vi "GUIAS POTÊNCIA VS VELOCIDADE.vi"() -> ()   [LabVIEW 2014]
uses:
  <vilib>/Platform/TimedLoop/XDataNode/timing_clust.ctl
  <vilib>/Platform/TimedLoop/XDataNode/nitl_modes.ctl
  <vilib>/Platform/TimedLoop/XDataNode/wakeup.ctl
  <vilib>/Instr/_visa.llb/VISA Configure Serial Port (Instr).vi
  <vilib>/Platform/TimedLoop/XDataNode/XDataNode.xnode
  <userlib>/Newport ESP301/Newport ESP301.lvlib
  <vilib>/Platform/TimedLoop/XDataNode/XDNodeRunTimeDep.lvlib
panel:
  in  "Refresh Button":bool
  out "XY Graph":cluster{dbl[], dbl[]}(graph)={[0.0, 0.0, 0.0, 0.0, 0.0, 0.0, 0.0, 0.0, 0.0, 0.0, 0.0, 0.0, 0.0, 0.0, 0.0, 0.0, 0.0, 0.0, 0.0, 0.0, 0.0, 0.0, 0.0, 0.0, 0.0, 0.0, 0.0, 0.0, 0.0, 0.0, 0.0, 0.0, 0.0, 0.0, 0.0, 0.0, 0.0, 0.0, 0.0, 0.0, 0.0, 0.0, 0.0, 0.0, 0.0, 0.0, 0.0, 0.0, 0.0, 0.0, 0.0, 0.0, 0.0, 0.0, 0.0, 0.0, 0.0, 0.0, 0.0, 0.0, 0.0, 0.0, 0.0, 0.0, 0.0, 0.0, 0.0, 0.0, 0.0, 0.0, 0.0, 0.0, 0.0, 0.0, 0.0, 0.0], [4600.0, 4600.0, 4600.0, 4600.0, 4600.0, 4600.0, 4600.0, 4600.0, 4600.0, 4600.0, 4600.0, 4600.0, 4600.0, 4600.0, 4600.0, 4600.0, 4600.0, 4600.0, 4600.0, 4600.0, 4600.0, 4600.0, 4600.0, 4600.0, 4600.0, 4600.0, 4600.0, 4690.0, 4802.5, 4800.5, 4799.5, 4799.5, 4799.5, 4800.0, 4800.0, 4800.0, 4800.0, 4800.0, 4800.0, 4800.0, 4800.0, 4800.0, 4800.0, 4800.0, 4995.5, 5001.5, 5000.5, 5000.0, 5000.0, 4999.5, 4999.5, 5000.0, 5000.0, 5000.0, 5000.0, 5000.0, 5000.0, 5000.0, 5000.0, 5000.0, 5000.0, 5000.0, 5000.0, 5000.0, 5000.0, 5000.0, 5000.0, 5000.0, 5000.0, 5000.0, 5000.0, 5000.0, 5000.0, 5000.0, 5000.0, 5000.0]}
  out "Y (um)":dbl format="%.1f"
  out "X (mm)":dbl format="%.2g"
  out "PROGRESSÃO":i32
  in  "DistGrupos":bool
  in  "dGroup":dbl=200.0
  in  "dGuia":dbl=100.0 format="%#_6f"
  in  "Iniciar":bool
  in  "Stop Button":bool
  in  "L":dbl=3.0 format="%.1f"
  in  "VELOCIDADES":dbl[](array[numeric])=[1.0, 5.0, 10.0, 20.0]
  in  "N_veloc":dbl=4.0
  # "Número de velocidades\npor potência"
  # "TAMANHO DA AMOSTRA (mm)"
  # "DISTÂNCIA ENTRE GUIAS (um)"
  # "DISTÂNCIA ENTRE GRUPOS (um)"
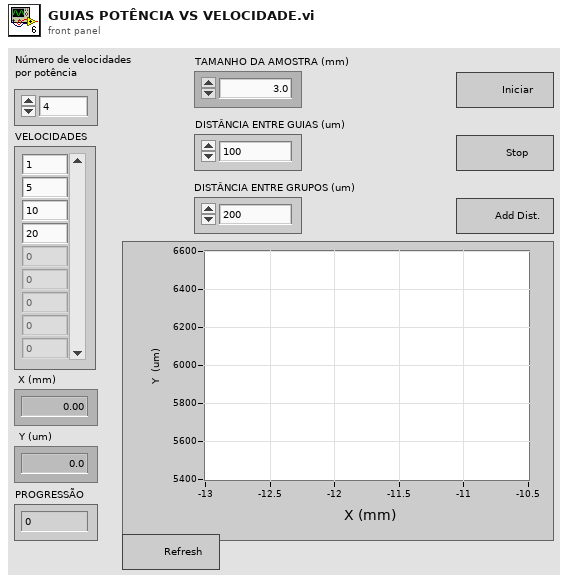
[diagram p1: front panel]
types:
  T1 = typedef "XDNodeRunTimeDep.lvlib/timing_clust.ctl" = cluster{"Expected End [f-1]":u64, "Actual End [f-1]":u64, "Finished Late? [f-1]":bool, "Expected End [i-1]":u64, "Actual End [i-1]":u64, "Finished Late? [i-1]":bool, "Expected Start [i]":u64, "Actual Start [i]":u64, "Expected Start [f]":u64, "Actual Start [f]":u64, "Source Name":string, "Structure Name":string, "Period":i64, "Deadline":i64, "Offset":i64, "Start":i64, "Priority":i32, "Timeout":i32, "Mode":T2, "Wakeup Reason":T3, "Error":errorcluster, "Source Type":string, "Secondary Source Type":string, "Global End Time":u64, "Global Start Time":u64, "Frame Duration":u64, "Iteration Duration":u64, "Assigned CPU":i32, "I/O Scan Engine Mode":u32}
  T2 = typedef "XDNodeRunTimeDep.lvlib/nitl_modes.ctl" = enum32{"No Change", "Process missed periods, maintain original phase", "Discard missed periods, maintain original phase", "Process missed periods, ignore original phase", "Discard missed periods, ignore original phase"}
  T3 = typedef "XDNodeRunTimeDep.lvlib/wakeup.ctl" = enum32{"Normal", "Aborted", "Asynchronous wakeup", "Timing source error", "Timed loop error", "Timeout"}
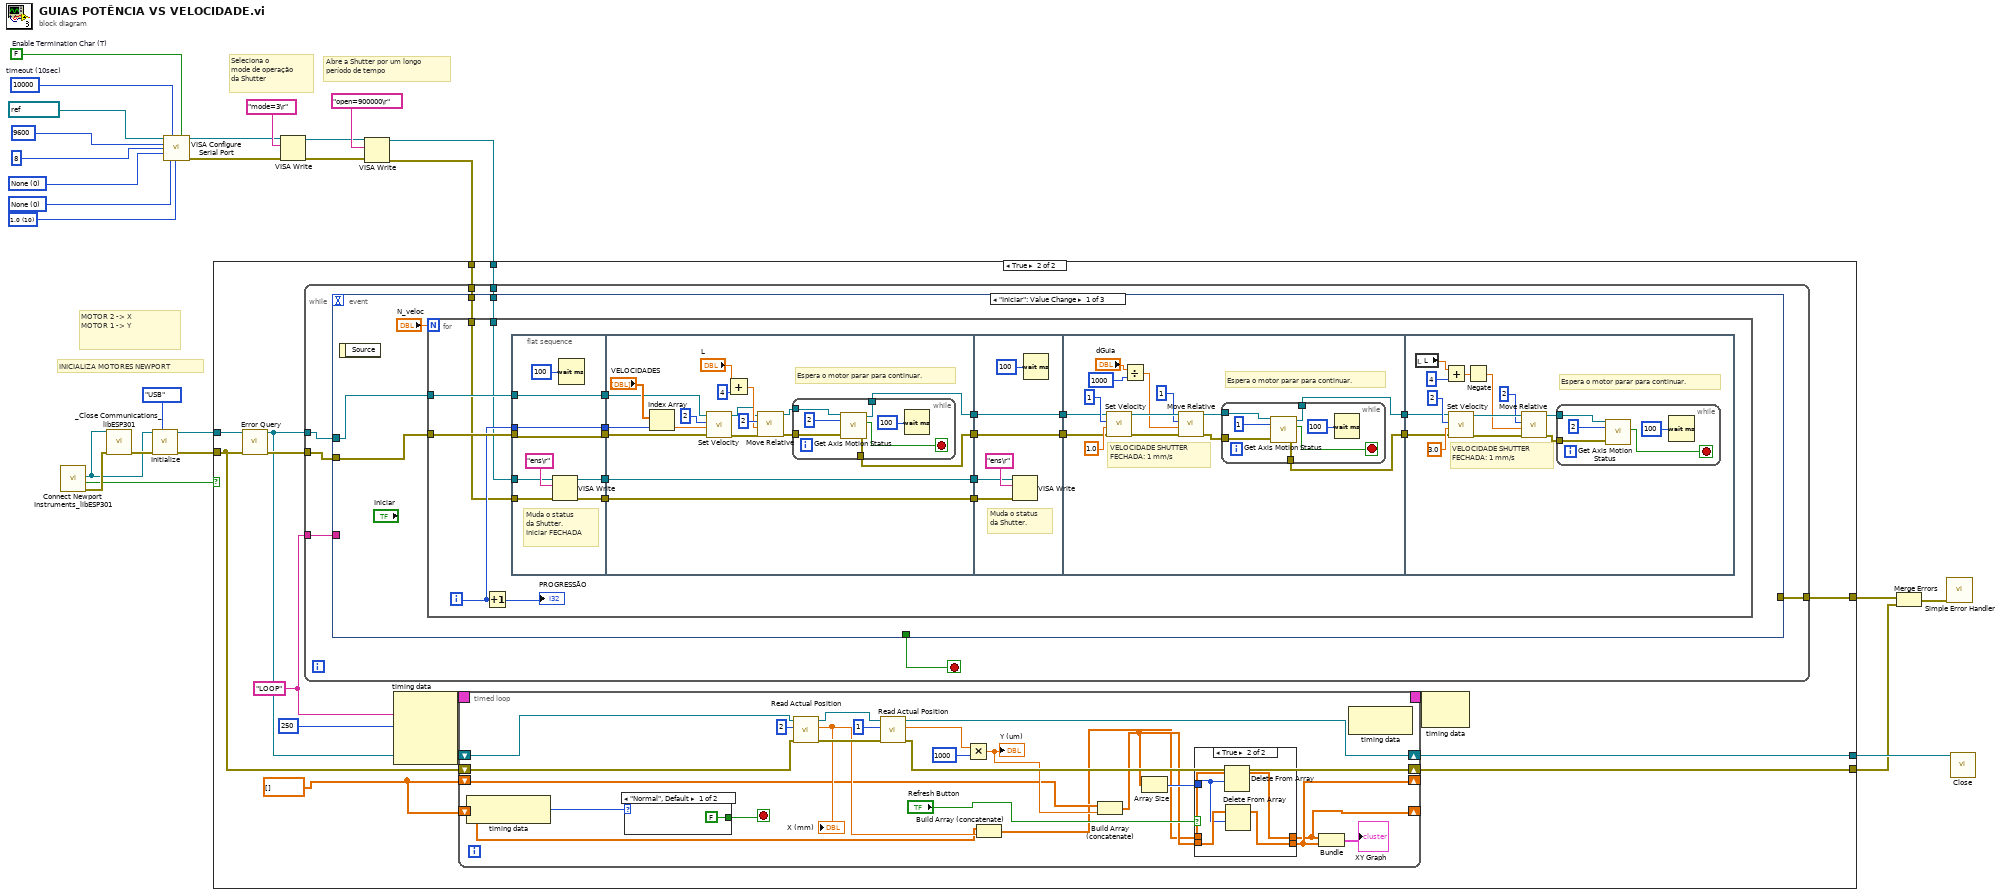
[diagram p0: block diagram]
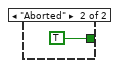
[diagram p4: hidden frame]
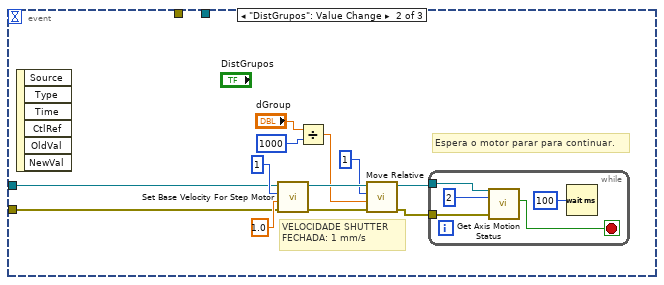
[diagram p5: hidden frame]
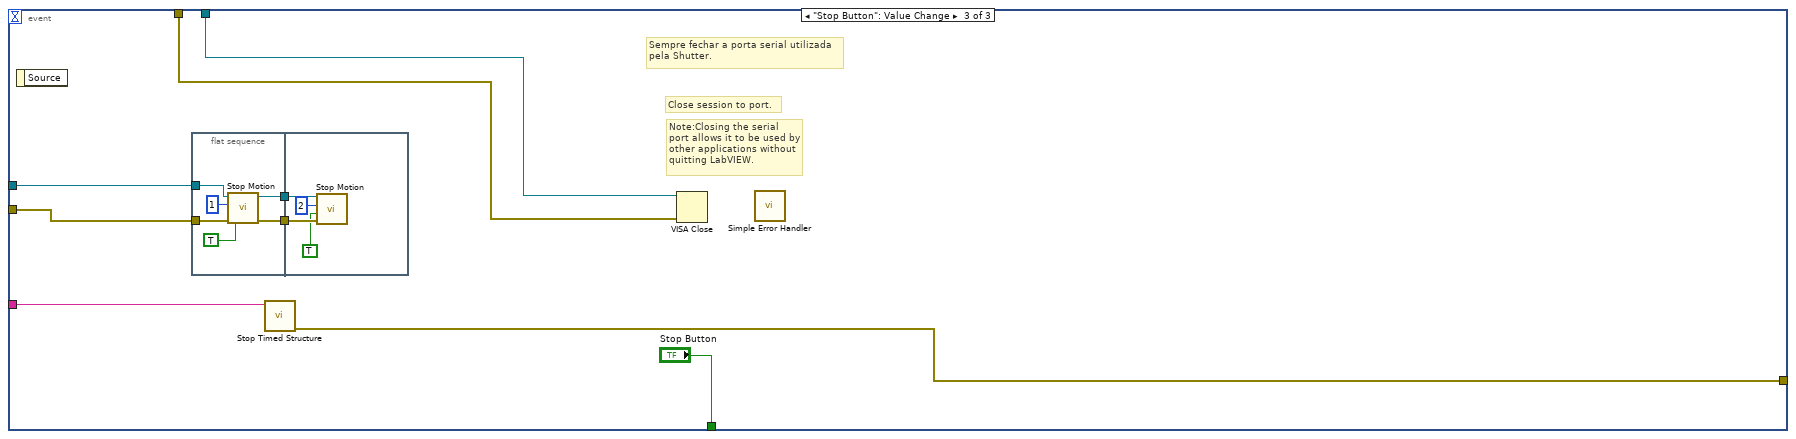
[diagram p6: hidden frame]
diagram:
  w15 = u16 0 items=["None", "Odd", "Even", "Mark", "Space"] ("parity")
  w18 = u16 10 items=["1.0"=10, "1.5"=15, "2.0"=20] ("stop bits")
  w19 = u16 0 items=["None"=0, "XON/XOFF"=1, "RTS/CTS"=2, "DTR/DSR"=4] ("flow control")
  w17 = FALSE  # Enable Termination Char (T)
  w16 = u32 10000  # timeout (10sec)
  # "MOTOR 2 -> X\nMOTOR 1 -> Y"
  # "Abre a Shutter por um longo\nperíodo de tempo"
  # "Seleciona o \nmode de operação\nda Shutter"
  # "INICIALIZA MOTORES NEWPORT"
  n1 = call <userlib>:"Connect Newport Instruments_libESP301.vi"() -> ("error (duplicate)"=w25:errorcluster, "Connected"=w23:bool, "VISA resource name (duplicate)"=w24:refnum<visa-resource-name>)  [unwired: 7 in, 2 out]
  n2 = call <userlib>:"_Close Communications_libESP301.vi"("Instrument Channel"=w24, "error in (no error)"=w25) -> ("error out"=w27:errorcluster)  [unwired: 13 in]
  n3 = call <userlib>:"Initialize.vi"("VISA resource name"=w24, "error in (no error)"=w27, "Serial Link (RS232)"=enum16{"RS232", "USB"}."USB") -> ("VISA resource name out"=w21:refnum<visa-resource-name>, "error out"=w22:errorcluster)  [unwired: 6 in]
  n4 = call-poly "VISA Configure Serial Port"("VISA resource name"=refnum<visa-resource-name> "COM6", "timeout (10sec)"=w16, "Enable Termination\nChar (T)"=w17, "baud rate (9600)"=u32 9600 ("baud rate"), "data bits (8)"=u16 8 ("data bits"), "parity (0:none)"=w15, "stop bits (10: 1 bit)"=w18, "flow control (0:none)"=w19) -> ("VISA resource name out"=w11:refnum<visa-resource-name>, "error out"=w10:errorcluster)  [unwired: 6 in]
  n5 = VISA Write(VISA resource name=w11, write buffer="mode=3\r", error in (no error)=w10) -> (VISA resource name out=w8:refnum<visa-resource-name>, error out=w7:errorcluster)  [unwired: 1 out]
  n6 = VISA Write(VISA resource name=w8, write buffer="open=900000\r", error in (no error)=w7) -> (VISA resource name out=w2:refnum<visa-resource-name>, error out=w1:errorcluster)  [unwired: 1 out]
  n7 = case shown="True" w23 {
    tunnel: w22 -> [w28 w39]
    tunnel: w21 -> [w29 w43]
    tunnel: [w29 w36] -> w6
    tunnel: [w28 w35] -> w4
    tunnel: [_ w33] -> w5
    tunnel: w2 -> [_ w32]
    tunnel: w1 -> [_ w31]
    frame False {
    }
    frame True {
      w30 = dbl[] []
      w34 = "LOOP" ("Structure Name")
      n8 = call <userlib>:"Error Query.vi"("error in (no error)"=w39, "VISA resource name"=w43) -> ("error out"=w42:errorcluster, "VISA resource name out"=w38:refnum<visa-resource-name>)  [unwired: 2 in, 2 out]
      n9 = while {
        tunnel: w38 -> [w90]
        tunnel: w42 -> [w89]
        tunnel: w34 -> [w87]
        tunnel: [w86] -> w33
        tunnel: w32 -> [w85]
        tunnel: w31 -> [w84]
        stop <- w88 stop-if-true
        n10 = event shown="[0] \"Iniciar\": Value Change" {
          selector: _ -> [_ _ _]
          dyn-events: _ -> [_ _ _]
          timeout: _ -> [_ _ _]
          tunnel: w90 -> [w93 w198 w217]
          tunnel: w89 -> [w94 w197 w216]
          tunnel: [_ _ "Stop Button"] -> w88
          tunnel: w87 -> [_ _ w214]
          tunnel: [_ _ w213] -> w86
          tunnel: w85 -> [w92 _ w212]
          tunnel: w84 -> [w91 _ w211]
          event "Iniciar": Value Change {
            n11 = event-data() -> ()  [unwired: 1 in, 1 out]
            n12 = for {
              N: "N_veloc" -> [_]
              tunnel: w94 -> [w114]
              tunnel: w93 -> [w113]
              tunnel: w92 -> [w98]
              tunnel: w91 -> [w97]
              i -> [w106]
              n13 = Increment(x=w106) -> (x+1=→"PROGRESSÃO":i32)
              n14 = flat-sequence {
                tunnel: w113 -> [w121]
                tunnel: w114 -> [w122]
                tunnel: w106 -> [w123]
                tunnel: [w123] -> w112
                tunnel: [w122] -> w111
                tunnel: [w121] -> w110
                tunnel: [w118] -> w109
                tunnel: [w117] -> w108
                tunnel: w98 -> [w116]
                tunnel: w97 -> [w115]
                tunnel: w112 -> [w141]
                tunnel: w111 -> [w129]
                tunnel: w110 -> [w128]
                tunnel: [w133] -> w104
                tunnel: w109 -> [w133]
                tunnel: w108 -> [w132]
                tunnel: [w132] -> w103
                tunnel: [w125] -> w101
                tunnel: [w124] -> w99
                tunnel: w104 -> [w152]
                tunnel: w103 -> [w151]
                tunnel: [w150] -> w102
                tunnel: w101 -> [w150]
                tunnel: [w149] -> w100
                tunnel: w99 -> [w149]
                tunnel: [w156] -> w107
                tunnel: w102 -> [w160]
                tunnel: w100 -> [w159]
                tunnel: [w155] -> w96
                tunnel: w107 -> [w179]
                tunnel: w96 -> [w178]
                frame #0 {
                  # "Muda o status\nda Shutter.\nIniciar FECHADA"
                  n15 = VISA Write(VISA resource name=w116, write buffer="ens\r", error in (no error)=w115) -> (VISA resource name out=w118:refnum<visa-resource-name>, error out=w117:errorcluster)  [unwired: 1 out]
                  n16 = Wait (ms)(milliseconds to wait=u32 100) -> ()  [unwired: 1 out]
                }
                frame #1 {
                  # "Espera o motor parar para continuar."
                  n17 = Index Array(array="VELOCIDADES", index=w141) -> (element=w134:dbl)
                  n18 = call <userlib>:"Set Velocity.vi"("error in (no error)"=w129, "Velocity (units/s)"=w134, "Axis (1)"=2, "VISA resource name"=w128) -> ("error out"=w130:errorcluster, "VISA resource name out"=w131:refnum<visa-resource-name>)  [unwired: 2 in]
                  n19 = Add(x="L", y=4) -> (x+y=w137:dbl)
                  n20 = call <userlib>:"Move Relative.vi"("error in (no error)"=w130, "Position (0 units)"=w137, "Axis (1)"=2, "VISA resource name"=w131) -> ("error out"=w127:errorcluster, "VISA resource name out"=w126:refnum<visa-resource-name>)  [unwired: 2 in]
                  n21 = while {
                    tunnel: [w145] -> w124
                    tunnel: [w144] -> w125
                    tunnel: w127 -> [w143]
                    tunnel: w126 -> [w142]
                    stop <- w147 stop-if-true
                    n22 = call <userlib>:"Get Axis Motion Status.vi"("error in (no error)"=w143, "Axis (1)"=2, "VISA resource name"=w142) -> ("error out"=w144:errorcluster, "Motion Done"=w147:bool, "VISA resource name out"=w145:refnum<visa-resource-name>)  [unwired: 2 in]
                    n23 = Wait (ms)(milliseconds to wait=u32 100) -> ()  [unwired: 1 out]
                  }
                }
                frame #2 {
                  # "Muda o status\nda Shutter."
                  n24 = VISA Write(VISA resource name=w152, write buffer="ens\r", error in (no error)=w151) -> ()  [unwired: 3 out]
                  n25 = Wait (ms)(milliseconds to wait=u32 100) -> ()  [unwired: 1 out]
                }
                frame #3 {
                  # "Espera o motor parar para continuar."
                  # "VELOCIDADE SHUTTER\nFECHADA: 1 mm/s"
                  n26 = call <userlib>:"Set Velocity.vi"("error in (no error)"=w160, "Velocity (units/s)"=1.0 ("Base Velocity (0 units/s)"), "Axis (1)"=1, "VISA resource name"=w159) -> ("error out"=w167:errorcluster, "VISA resource name out"=w166:refnum<visa-resource-name>)  [unwired: 2 in]
                  n27 = Divide(x="dGuia", y=1000) -> (x/y=w161:dbl)
                  n28 = call <userlib>:"Move Relative.vi"("error in (no error)"=w167, "Position (0 units)"=w161, "Axis (1)"=1, "VISA resource name"=w166) -> ("error out"=w157:errorcluster, "VISA resource name out"=w158:refnum<visa-resource-name>)  [unwired: 2 in]
                  n29 = while {
                    tunnel: [w172] -> w156
                    tunnel: [w171] -> w155
                    tunnel: w157 -> [w170]
                    tunnel: w158 -> [w169]
                    stop <- w174 stop-if-true
                    n30 = call <userlib>:"Get Axis Motion Status.vi"("error in (no error)"=w170, "Axis (1)"=1, "VISA resource name"=w169) -> ("error out"=w171:errorcluster, "Motion Done"=w174:bool, "VISA resource name out"=w172:refnum<visa-resource-name>)  [unwired: 2 in]
                    n31 = Wait (ms)(milliseconds to wait=u32 100) -> ()  [unwired: 1 out]
                  }
                }
                frame #4 {
                  # "Espera o motor parar para continuar."
                  # "VELOCIDADE SHUTTER\nFECHADA: 1 mm/s"
                  n32 = local read "L"() -> (w182:dbl)
                  n33 = Add(x=w182, y=4) -> (x+y=w181:dbl)
                  n34 = call <userlib>:"Set Velocity.vi"("error in (no error)"=w178, "Velocity (units/s)"=3.0 ("Base Velocity (0 units/s)"), "Axis (1)"=2, "VISA resource name"=w179) -> ("error out"=w187:errorcluster, "VISA resource name out"=w186:refnum<visa-resource-name>)  [unwired: 2 in]
                  n35 = Negate(x=w181) -> (-x=w180:dbl)
                  n36 = call <userlib>:"Move Relative.vi"("error in (no error)"=w187, "Position (0 units)"=w180, "Axis (1)"=2, "VISA resource name"=w186) -> ("error out"=w176:errorcluster, "VISA resource name out"=w177:refnum<visa-resource-name>)  [unwired: 2 in]
                  n37 = while {
                    tunnel: w176 -> [w190]
                    tunnel: w177 -> [w189]
                    stop <- w192 stop-if-true
                    n38 = call <userlib>:"Get Axis Motion Status.vi"("error in (no error)"=w190, "Axis (1)"=2, "VISA resource name"=w189) -> ("Motion Done"=w192:bool)  [unwired: 2 in, 2 out]
                    n39 = Wait (ms)(milliseconds to wait=u32 100) -> ()  [unwired: 1 out]
                  }
                }
              }
            }
          }
          event "DistGrupos": Value Change {
            # "Espera o motor parar para continuar."
            # "VELOCIDADE SHUTTER\nFECHADA: 1 mm/s"
            n40 = event-data() -> ()  [unwired: 1 in, 6 out]
            n41 = call <userlib>:"Set Base Velocity For Step Motor.vi"("error in (no error)"=w197, "Base Velocity (0 units/s)"=1.0, "Axis (1)"=1, "VISA resource name"=w198) -> ("error out"=w204:errorcluster, "VISA resource name out"=w203:refnum<visa-resource-name>)  [unwired: 2 in]
            n42 = Divide(x="dGroup", y=1000) -> (x/y=w199:dbl)
            n43 = call <userlib>:"Move Relative.vi"("error in (no error)"=w204, "Position (0 units)"=w199, "Axis (1)"=1, "VISA resource name"=w203) -> ("error out"=w194:errorcluster, "VISA resource name out"=w195:refnum<visa-resource-name>)  [unwired: 2 in]
            n44 = while {
              tunnel: w194 -> [w207]
              tunnel: w195 -> [w206]
              stop <- w209 stop-if-true
              n45 = call <userlib>:"Get Axis Motion Status.vi"("error in (no error)"=w207, "Axis (1)"=2, "VISA resource name"=w206) -> ("Motion Done"=w209:bool)  [unwired: 2 in, 2 out]
              n46 = Wait (ms)(milliseconds to wait=u32 100) -> ()  [unwired: 1 out]
            }
          }
          event "Stop Button": Value Change {
            # "Sempre fechar a porta serial utilizada\npela Shutter."
            # "Note:Closing the serial port allows it to be used by other applications without\nquitting LabVIEW."
            # "Close session to port."
            n47 = event-data() -> ()  [unwired: 1 in, 1 out]
            n48 = flat-sequence {
              tunnel: w217 -> [w225]
              tunnel: w216 -> [w224]
              tunnel: [w222] -> w219
              tunnel: [w221] -> w218
              tunnel: w219 -> [w229]
              tunnel: w218 -> [w228]
              frame #0 {
                n49 = call <userlib>:"Stop Motion.vi"("error in (no error)"=w224, "Stop all axes (F)"=TRUE, "Axis (1)"=1, "VISA resource name"=w225) -> ("error out"=w221:errorcluster, "VISA resource name out"=w222:refnum<visa-resource-name>)  [unwired: 2 in]
              }
              frame #1 {
                n50 = call <userlib>:"Stop Motion.vi"("error in (no error)"=w228, "Stop all axes (F)"=TRUE, "Axis (1)"=2, "VISA resource name"=w229) -> ()  [unwired: 2 in, 2 out]
              }
            }
            n51 = call <vilib>:"Stop Timed Structure.vi"("name"=w214) -> ("error out"=w213:errorcluster)  [unwired: 10 in]
            n52 = VISA Close(VISA resource name=w212, error in (no error)=w211) -> ()  [unwired: 1 out]
            n53 = call <vilib>:"Simple Error Handler.vi"() -> ()  [unwired: 5 in, 5 out]
          }
        }
      }
      n54 = node-c288(w34, i64 250 ("Period")) -> (w41:T1)  [unwired: 2 in]
      n55 = timed-loop {
        timing: w41 -> [_]
        timing-out: [_] -> w40
        shift-right: [w60] -> w36
        shift-left: w38 -> [w65]
        shift-right: [w59] -> w35
        shift-left: w39 -> [w64]
        shift-right: [w45] -> _
        shift-left: w30 -> [w49]
        shift-right: [w44] -> _
        shift-left: w30 -> [w47]
        stop <- w57 stop-if-true
        n56 = node-c288() -> (w58:T3)  [unwired: 1 in]
        n57 = case shown="\"Normal\", Default" w58 {
          tunnel: [FALSE TRUE] -> w57
          frame "Normal", Default {
          }
          frame "Aborted" {
          }
        }
        n58 = call <userlib>:"Read Actual Position.vi"("error in (no error)"=w64, "Axis (1)"=2, "VISA resource name"=w65) -> ("error out"=w63:errorcluster, "Position (units)"=w56:dbl, "VISA resource name out"=w62:refnum<visa-resource-name>)  [unwired: 2 in]
        "X (mm)" <- w56
        n59 = call <userlib>:"Read Actual Position.vi"("error in (no error)"=w63, "Axis (1)"=1, "VISA resource name"=w62) -> ("error out"=w59:errorcluster, "Position (units)"=w53:dbl, "VISA resource name out"=w60:refnum<visa-resource-name>)  [unwired: 2 in]
        n60 = Multiply(x=w53, y=u32 1000) -> (x*y=w52:dbl)
        "Y (um)" <- w52
        n61 = Build Array (concatenate)(w47, w56) -> (w46:dbl[])
        n62 = Build Array (concatenate)(w49, w52) -> (w48:dbl[])
        n63 = Array Size(array=w48) -> (size(s)=w50:i32)
        n64 = case shown="True" "Refresh Button" {
          tunnel: [w68 w70] -> w44
          tunnel: w46 -> [w68 w73]
          tunnel: [w67 w69] -> w45
          tunnel: w48 -> [w67 w72]
          tunnel: w50 -> [_ w71]
          frame False {
          }
          frame True {
            n65 = Delete From Array(array=w73, length=w71) -> (array with subset deleted=w70:dbl[])  [unwired: 1 in, 1 out]
            n66 = Delete From Array(array=w72, length=w71) -> (array with subset deleted=w69:dbl[])  [unwired: 1 in, 1 out]
          }
        }
        n67 = Bundle(w44, w45) -> (→"XY Graph":cluster{dbl[], dbl[]})  [unwired: 1 in]
        n68 = node-c288() -> ()  [unwired: 1 in, 1 out]
      }
      n69 = node-c288(w40) -> ()  [unwired: 1 out]
    }
  }
  n70 = Merge Errors(w5, w4) -> (w3:errorcluster)
  n71 = call <vilib>:"Simple Error Handler.vi"("error in (no error)"=w3) -> ()  [unwired: 1 in, 8 out]
  n72 = call <userlib>:"Close.vi"("VISA resource name"=w6) -> ()  [unwired: 10 in, 1 out]
